vi "Creators Is Created Queue.vi"(10 "Created Queue Alias":string, 11 "Template Event in":refnum<class "Template Event.lvclass">) -> (2 "Is Created Queue?":bool, 3 "Template Event out":refnum<class "Template Event.lvclass">)   [LabVIEW 2021, in "_Template.lvlib" / "Templates.lvlib" / "Template Event.lvlib" / "Template Event.lvclass"]
uses:
  Template Event.lvclass
  Template Event.lvclass/Template Event.ctl
  <vilib>/jettl/jettl/jettl/Event/Event.lvclass
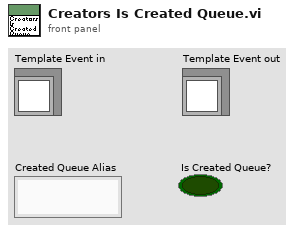
[diagram p1: front panel]
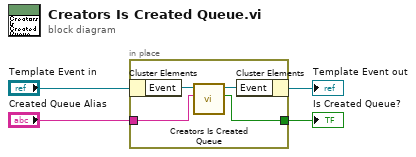
[diagram p0: block diagram]
diagram:
  n1 = in-place {
    in-place-border: [w6] -> w2
    in-place-border: "Created Queue Alias" -> [w5]
    n2 = in-place-cluster #1("Template Event in") -> ("Event"=w8:refnum<class "Event.lvclass">)
    n3 = call-dynamic "Creators Is Created Queue.vi"("Created Queue Alias"=w5, "Event in"=w8) -> ("Is Created Queue?"=w6:bool, "Event out"=w7:refnum<class "Event.lvclass">)  [unwired: 8 in]
    n4 = in-place-cluster #1("Event"=w7) -> (→"Template Event out":refnum<class "Template Event.lvclass">)
  }
  "Is Created Queue?" <- w2
